vi "SJ_Get_Signal_Phase.vi"(8 "No of Analogue Samples":i32=600, 9 "Number of Cycles":i32=1, 10 "Actual Sampling Frequency":dbl=12000.0, 11 "Signal":dbl[](array[numeric])) -> (3 "Phase Angle _deg_":dbl)   [LabVIEW 2011]
uses:
  <vilib>/Analysis/2dsp.llb/1D Cross Correlation (DBL).vi
  <vilib>/Analysis/NI_AALBase.lvlib
  <vilib>/Analysis/NI_AALPro.lvlib
  <vilib>/Analysis/NI_AAL_SigProc.lvlib
panel:
  out "Waveform Graph":dbl[](graph)
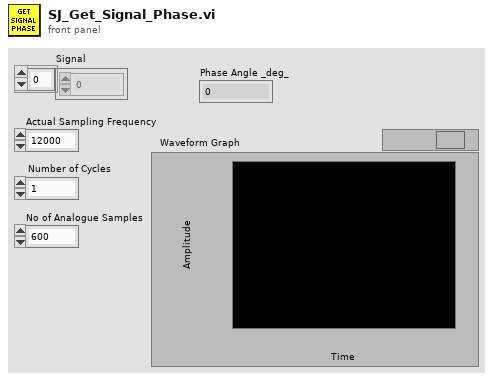
[diagram p1: front panel]
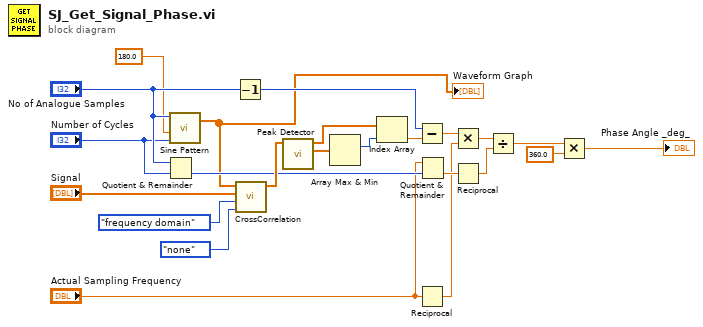
[diagram p0: block diagram]
diagram:
  n1 = Quotient & Remainder(x="No of Analogue Samples", y="Number of Cycles") -> (floor(x/y)=w17:i32)  [unwired: 1 out]
  n2 = call <vilib>:"Sine Pattern.vi"("cycles"="Number of Cycles", "phase(degrees)"=180.0, "samples"="No of Analogue Samples") -> ("Sinusoidal Pattern"=w2:dbl[])  [unwired: 1 in, 1 out]
  "Waveform Graph" <- w2
  n3 = Decrement(x="No of Analogue Samples") -> (x-1=w7:i32)
  n4 = call-poly <vilib>:"CrossCorrelation.vi"("normalization"=enum32{"none", "unbiased", "biased"}."none", "algorithm"=enum32{"direct", "frequency domain"}."frequency domain", "Y"="Signal", "X"=w2) -> ("Rxy"=w22:dbl[])  [unwired: 6 in, 1 out]
  n5 = call <vilib>:"Peak Detector.vi"("X"=w22) -> ("Amplitudes"=w21:dbl[], "Locations"=w20:dbl[])  [unwired: 6 in, 3 out]
  n6 = Array Max & Min(array=w21) -> (max index (indices)=w19:i32)  [unwired: 3 out]
  n7 = Index Array(array=w20, index=w19) -> (element=w6:dbl)
  n8 = Subtract(x=w7, y=w6) -> (x-y=w14:dbl)
  n9 = Reciprocal(x="Actual Sampling Frequency") -> (1/x=w13:dbl)
  n10 = Quotient & Remainder(x="Actual Sampling Frequency", y=w17) -> (floor(x/y)=w15:dbl)  [unwired: 1 out]
  n11 = Multiply(x=w14, y=w13) -> (x*y=w11:dbl)
  n12 = Reciprocal(x=w15) -> (1/x=w12:dbl)
  n13 = Divide(x=w11, y=w12) -> (x/y=w10:dbl)
  n14 = Multiply(x=w10, y=360.0) -> (x*y=→"Phase Angle _deg_":dbl)
